vi "HEWH Gas Thermal Raw Calc.vi"(1 "Use Constant Thermal Efficiency":bool, 2 "Gas Mass Flow":dbl, 3 "Gas Totalizer":dbl format="%#_13g", 5 "RTD Out (Deg F)":dbl, 7 "Constant Thermal Eff":dbl format="%#.5g", 9 "RTD In (Deg F)":dbl, 11 "error in (no error)":errorcluster, 12 "Gallons (Gal)":dbl, 14 "Gross Heating Value, Vol (Real, Dry)":dbl) -> (4 "Rate":dbl, 6 "Eff":dbl format="%#.5g", 15 "error out":errorcluster)   [LabVIEW 2020]
uses:
  HEWH Water Properties.ctl
panel:
  out "B":dbl
  out "A":dbl
  out "Heat input":dbl
  # "Common Parameters"
  # "Real Time Calculation of Thermal (False)"
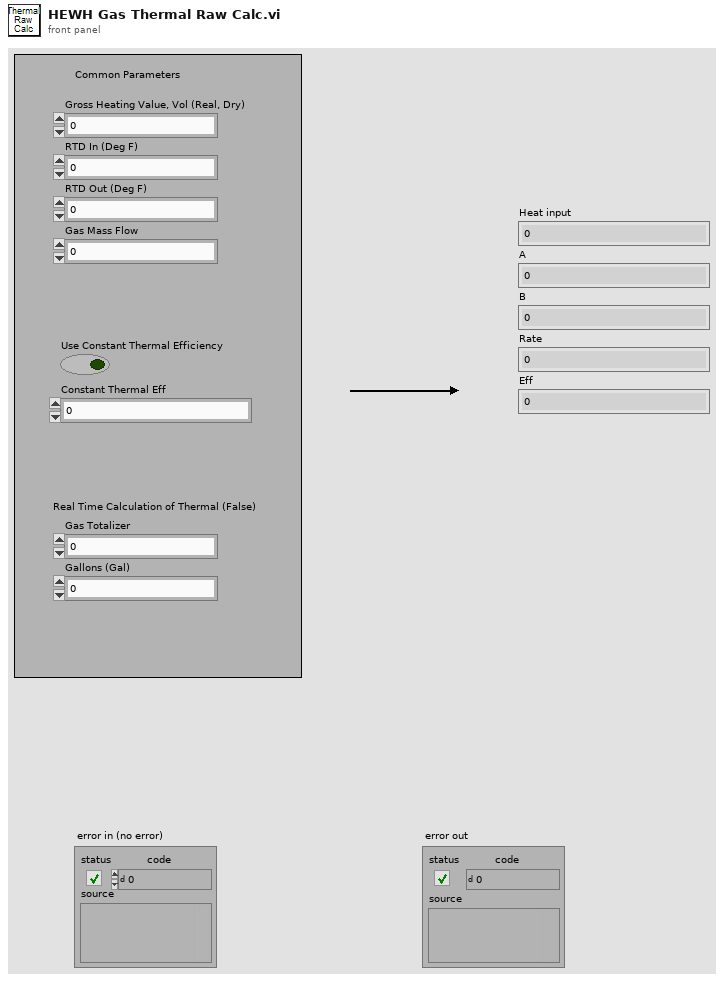
[diagram p1: front panel]
types:
  T1 = typedef "HEWH Water Properties.ctl" = enum16{"GEA Intertek Values", "CSA Values", "ANSI Values"}
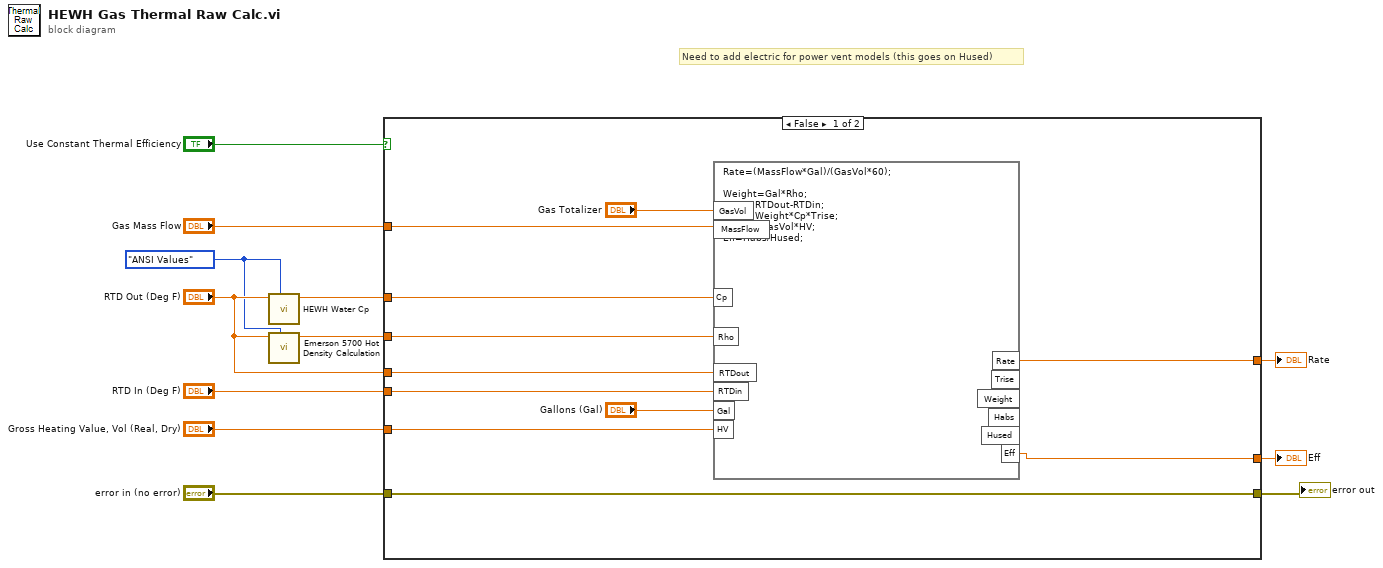
[diagram p0: block diagram]
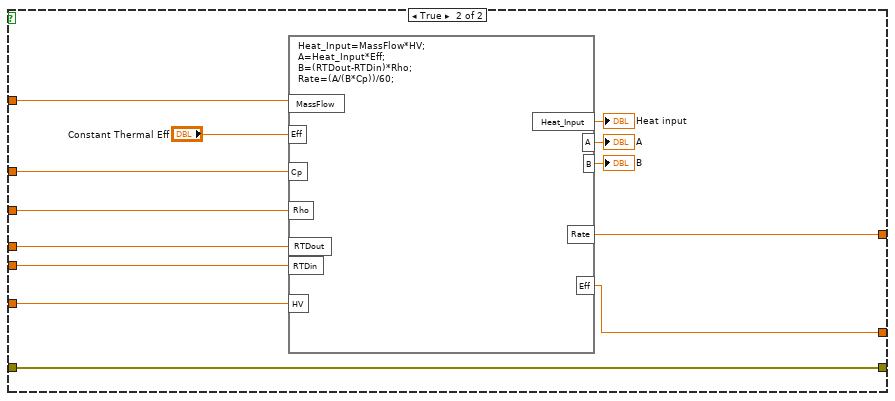
[diagram p2: hidden frame]
diagram:
  w6 = HEWH_Water_Properties."ANSI Values" ("Water Properties Reference")
  # "Need to add electric for power vent models (this goes on Hused)"
  n1 = call "HEWH Water Cp.vi"("Water Properties Reference"=w6, "Input Temperature (°F)"="RTD Out (Deg F)") -> ("Specific Heat (BTU/lbm*F)"=w7:dbl)  [unwired: 8 in, 1 out]
  n2 = call "Emerson 5700 Hot Density Calculation.vi"("Water Properties Reference"=w6, "RTD Out (°F)"="RTD Out (Deg F)") -> ("Density (lb/gal)"=w8:dbl)  [unwired: 8 in, 1 out]
  n3 = case shown="False" "Use Constant Thermal Efficiency" {
    tunnel: [w21 w36] -> w12
    tunnel: "error in (no error)" -> [w21 w36]
    tunnel: "RTD Out (Deg F)" -> [w20 w34]
    tunnel: w8 -> [w19 w30]
    tunnel: w7 -> [w18 w31]
    tunnel: "RTD In (Deg F)" -> [w17 w35]
    tunnel: "Gross Heating Value, Vol (Real, Dry)" -> [w16 w33]
    tunnel: "Gas Mass Flow" -> [w15 w32]
    tunnel: [w14 w28] -> w2
    tunnel: [w13 w24] -> w1
    frame False {
      n4 = formula code="Rate=(MassFlow*Gal)/(GasVol*60);\n\nWeight=Gal*Rho;\nTrise=RTDout-RTDin;\nHabs=Weight*Cp*Trise;\nHused=GasVol*HV;\nEff=Habs/Hused;"("RTDout"=w20, "RTDin"=w17, "MassFlow"=w15, "Gal"="Gallons (Gal)", "GasVol"="Gas Totalizer", "HV"=w16, "Cp"=w18, "Rho"=w19) -> ("Rate"=w14:dbl, "Eff"=w13:dbl)  [unwired: 4 out]
    }
    frame True {
      n5 = formula code="Heat_Input=MassFlow*HV;\nA=Heat_Input*Eff;\nB=(RTDout-RTDin)*Rho;\nRate=(A/(B*Cp))/60;"("RTDout"=w34, "RTDin"=w35, "MassFlow"=w32, "HV"=w33, "Cp"=w31, "Rho"=w30, "Eff"="Constant Thermal Eff") -> ("Rate"=w28:dbl, "Heat_Input"=→"Heat input":dbl, "A"=→"A":dbl, "B"=→"B":dbl, "Eff"=w24:dbl)
    }
  }
  "error out" <- w12
  "Rate" <- w2
  "Eff" <- w1
